vi "Receive Read Data Response.vi"(8 "error in (no error)":errorcluster, 11 "Port Selection Info":T1={"Port Name"="", "Amplifier Num"=1, "Baud Rate"=38400, "Char Formation"=enum."0"} {"Baud Rate" items=["38400"=38400, "19200"=19200, "9600"=9600, "115200"=0]; "Amplifier Num" max=31}) -> (0 "error out":errorcluster, 1 "Data":u32[](array[numeric]), 2 "byte num":u8, 3 "Port Selection Info Out":T1={"Port Name"="", "Amplifier Num"=1, "Baud Rate"=38400, "Char Formation"=enum."0"} {"Baud Rate" items=["38400"=38400, "19200"=19200, "9600"=9600, "115200"=0]; "Amplifier Num" max=31}, 4 "CRC Match":bool, 5 "FC":u8, 7 "Bank":u8)   [LabVIEW 2014, in "ALPHA5 RS485.lvlib"]
uses:
  ALPHA5 RS485.lvlib
  typedefs/Port Selection Info.ctl
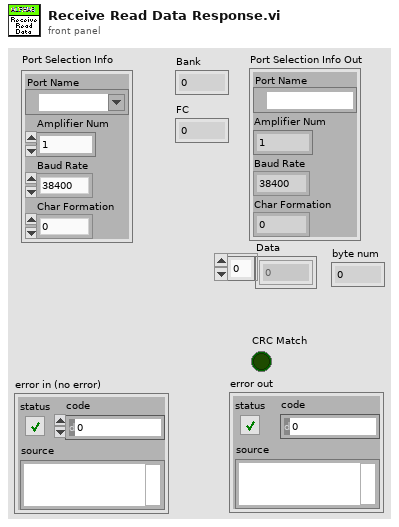
[diagram p1: front panel]
types:
  T1 = typedef "ALPHA5 RS485.lvlib/Port Selection Info.ctl" = cluster{"Port Name":refnum<visa-resource-name>, "Amplifier Num":u8, "Baud Rate":u32, "Char Formation":enum16{"0", "1", "2", "3", "4", "5"}}
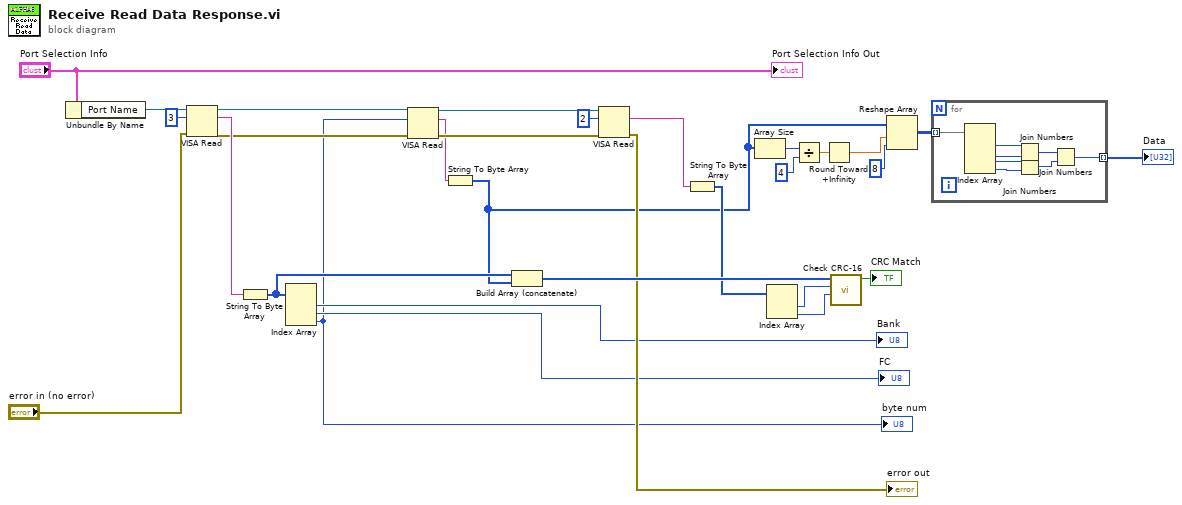
[diagram p0: block diagram]
diagram:
  n1 = Unbundle By Name("Port Selection Info") -> ("Port Name"=w29:refnum<visa-resource-name>)
  n2 = VISA Read(VISA resource name=w29, byte count=u32 3, error in (no error)="error in (no error)") -> (VISA resource name out=w25:refnum<visa-resource-name>, read buffer=w26:string, error out=w24:errorcluster)  [unwired: 1 out]
  n3 = String To Byte Array(string=w26) -> (unsigned byte array=w20:u8[])
  n4 = Index Array(array=w20) -> (element #1=→"Bank":u8, element #2=→"FC":u8, element #3=w9:u8)  [unwired: 3 in]
  "byte num" <- w9
  n5 = VISA Read(VISA resource name=w25, byte count=w9, error in (no error)=w24) -> (VISA resource name out=w23:refnum<visa-resource-name>, read buffer=w19:string, error out=w22:errorcluster)  [unwired: 1 out]
  n6 = String To Byte Array(string=w19) -> (unsigned byte array=w5:u8[])
  n7 = Build Array (concatenate)(w20, w5) -> (w18:u8[])
  n8 = VISA Read(VISA resource name=w23, byte count=u32 2, error in (no error)=w22) -> (read buffer=w17:string, error out=→"error out":errorcluster)  [unwired: 2 out]
  n9 = String To Byte Array(string=w17) -> (unsigned byte array=w16:u8[])
  n10 = Array Size(array=w5) -> (size(s)=w8:i32)
  n11 = Index Array(array=w16) -> (element #1=w14:u8, element #2=w15:u8)  [unwired: 2 in]
  n12 = Divide(x=w8, y=4) -> (x/y=w6:dbl)
  n13 = Round Toward +Infinity(x=w6) -> (ceil(x): smallest int >= x=w4:dbl)
  n14 = call "Check CRC-16.vi"("CRC-16-H"=w15, "CRC-16-L"=w14, "Data In"=w18) -> ("Check Result"=→"CRC Match":bool)  [unwired: 7 in, 1 out]
  n15 = Reshape Array(w5, w4, 8 ("dimension size")) -> (w2:u8[][])
  n16 = for {
    tunnel: w2 -> [w32] mode=indexing
    tunnel: [w31] -> w1 mode=indexing
    n17 = Index Array(array=w32) -> (element #1=w38:u8, element #2=w37:u8, element #3=w36:u8, element #4=w35:u8)  [unwired: 4 in]
    n18 = Join Numbers(hi=w38, lo=w37) -> ((hi.lo)=w34:u16)
    n19 = Join Numbers(hi=w36, lo=w35) -> ((hi.lo)=w33:u16)
    n20 = Join Numbers(hi=w34, lo=w33) -> ((hi.lo)=w31:u32)
  }
  "Data" <- w1
  "Port Selection Info Out" <- "Port Selection Info"
